vi "Reset graph and table.vi"(4 "Error in":errorcluster, 7 "App state":T1) -> (0 "Error out":errorcluster, 3 "App state":T1)   [LabVIEW 2020]
uses:
  Global variables/Control and indicators refs.vi
  Typedefs/State.ctl
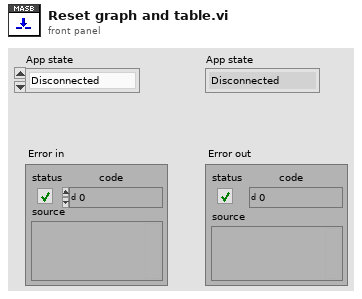
[diagram p1: front panel]
types:
  T1 = typedef "State.ctl" = enum16{"Disconnected", "Connected", "Measuring"}
  T2 = typedef "Control and indicators refs.ctl" = cluster{"Device":refnum<vi>, "Connect":refnum<vi>, "Measurement":refnum<vi>, "CV configuration":refnum<vi>, "I-V Graph":refnum<vi>}
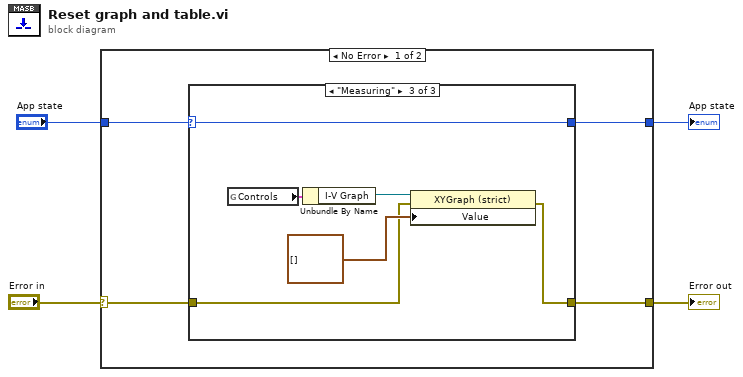
[diagram p0: block diagram]
diagram:
  n1 = case shown="No Error" "Error in" {
    selector: "Error in" -> [w6 w20]
    tunnel: [w5 w20] -> w3
    tunnel: "App state" -> [w8 w19]
    tunnel: [w7 w19] -> w1
    frame No Error {
      n2 = case shown="\"Measuring\"" w8 {
        selector: w8 -> [w9 w12 w13]
        tunnel: [w9 w12 w13] -> w7
        tunnel: w6 -> [w10 w11 w15]
        tunnel: [w10 w11 w14] -> w5
        frame "Disconnected", Default {
        }
        frame "Connected" {
        }
        frame "Measuring" {
          n3 = global read "Control and indicators refs.vi" "Controls"() -> (w18:T2)
          n4 = Unbundle By Name(w18) -> ("I-V Graph"=w17:refnum<vi>)
          n5 = property class="XYGraph (strict)"(reference=w17, error in=w15, "Value"=cluster{"X":dbl, "Y":dbl}[] []) -> (error out=w14:errorcluster)  [unwired: 1 out]
        }
      }
    }
    frame Error {
    }
  }
  "Error out" <- w3
  "App state" <- w1
